vi "Factor escala.vi"(11 "Entrada":dbl) -> (3 "Numeric":dbl)   [LabVIEW 2019]
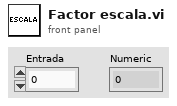
[diagram p1: front panel]
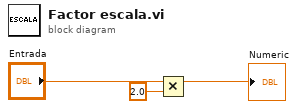
[diagram p0: block diagram]
diagram:
  n1 = Multiply(x="Entrada", y=2.0) -> (x*y=→"Numeric":dbl)
